vi "IDS_SubMasterExample_ErrorMessage.vi"(4 "Error":errorcluster, 10 "String in":refnum<vi>) -> ()   [LabVIEW 2016]
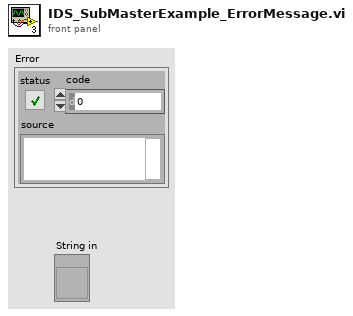
[diagram p1: front panel]
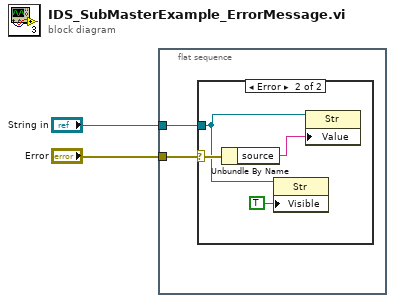
[diagram p0: block diagram]
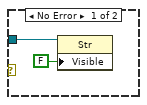
[diagram p2: hidden frame]
diagram:
  n1 = flat-sequence {
    tunnel: "String in" -> [w4]
    tunnel: "Error" -> [w3]
    frame #0 {
      n2 = case shown="Error" w3 {
        selector: w3 -> [_ w10]
        tunnel: w4 -> [w6 w8]
        frame No Error {
          n3 = property class="Str"(reference=w6, "Visible"=FALSE) -> ()  [unwired: 1 in, 2 out]
        }
        frame Error {
          n4 = Unbundle By Name(w10) -> ("source"=w9:string)
          n5 = property class="Str"(reference=w8, "Visible"=TRUE) -> ()  [unwired: 1 in, 2 out]
          n6 = property class="Str"(reference=w8, "Value"=w9) -> ()  [unwired: 1 in, 2 out]
        }
      }
    }
  }
